vi "Logger Started.vi"(8 "error in (no error)":errorcluster, 10 "Logger Started":T1, 11 "Historian Logger in":refnum<class "Historian Logger.lvclass">) -> (0 "error out":errorcluster, 3 "Historian Logger out":refnum<class "Historian Logger.lvclass">)   [LabVIEW 2020, in "VolatusHistorian.lvlib" / "Historian Logger.lvclass"]
uses:
  Historian Logger.lvclass
  Historian Logger.lvclass/Historian Logger.ctl
  VolatusData/Logger State.ctl
  VolatusData/VolatusData.lvlib
  VolatusData/Logger Started.ctl
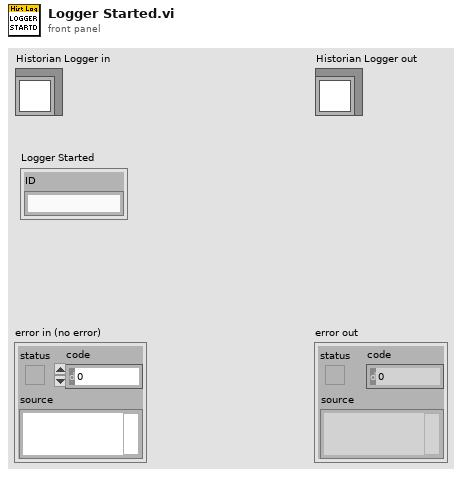
[diagram p1: front panel]
types:
  T1 = typedef "VolatusData.lvlib/Logger Started.ctl" = cluster{"ID":string}
  T2 = typedef "VolatusData.lvlib/Logger State.ctl" = enum16{"Unknown", "Idle", "Preparing", "Ready", "Logging", "Stopping"}
  T3 = typedef "VolatusHistorian.lvlib/Historian Logger.lvclass/Group Info.ctl" = cluster{"Buffer":refnum<class "Group Buffer DBL.lvclass">, "Logger":refnum<class "MessageQ.lvclass">, "Group":refnum<class "Group DBL.lvclass">, "Last Timestamp":dbl, "State":T2}
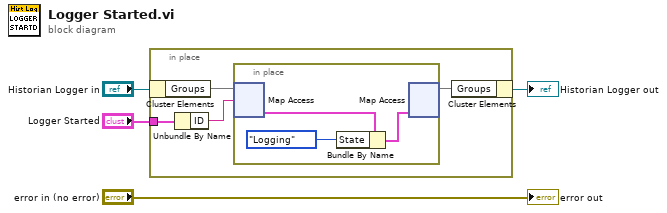
[diagram p0: block diagram]
diagram:
  n1 = in-place {
    in-place-border: "Logger Started" -> [w8]
    n2 = in-place-cluster #1("Historian Logger in") -> ("Groups"=w7:map{string, T3})
    n3 = Unbundle By Name(w8) -> ("ID"=w6:string)
    n4 = in-place {
      n5 = in-place-map #2(w7, w6) -> (w9:T3)  [unwired: 1 in, 1 out]
      n6 = Bundle By Name(cluster=w9, "State"=Logger_State."Logging") -> (w10:T3)
      n7 = in-place-map #2(w10) -> (w5:map{string, T3})  [unwired: 1 in, 2 out]
    }
    n8 = in-place-cluster #1("Groups"=w5) -> (→"Historian Logger out":refnum<class "Historian Logger.lvclass">)
  }
  "error out" <- "error in (no error)"
